vi "dfd_Lattice to Normalized Lattice.vi"(11 "k [M~1]":dbl[](array[numeric]) format="%.2f") -> (3 "k & ^k":dbl[](array[numeric]) format="%.2f")   [LabVIEW 2017, in "NI_DigFilterLicensed.lvlib"]
uses:
  <vilib>/addons/Digital Filter Design/NI_DigFilterLicensed.lvlib
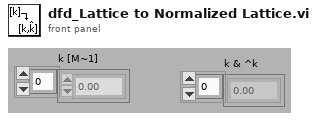
[diagram p1: front panel]
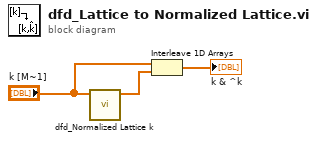
[diagram p0: block diagram]
diagram:
  n1 = call <vilib>:"dfd_Normalized Lattice k.vi"("k"="k [M~1]") -> ("^k"=w3:dbl[])  [unwired: 10 out]
  n2 = Interleave 1D Arrays("k [M~1]", w3) -> (→"k & ^k":dbl[])
